vi "DAQmx task start-Pockels modulation AO.vi"(8 "error in (no error)":errorcluster, 11 "Pockels modulation AO task in":refnum<k21>) -> (0 "error out":errorcluster, 3 "Pockels modulation AO task out":refnum<k21>)   [LabVIEW 2020]
uses:
  Globals/gl_Pockels control globals.vi
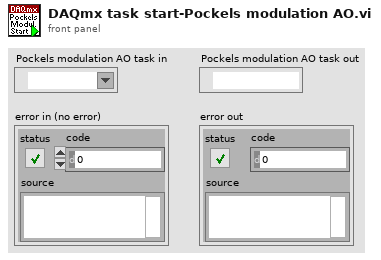
[diagram p1: front panel]
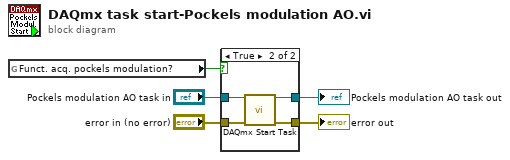
[diagram p0: block diagram]
diagram:
  n1 = global read "gl_Pockels control globals.vi" "Funct. acq. pockels modulation?"() -> (w4:bool)
  n2 = case shown="True" w4 {
    tunnel: [w6 w10] -> w1
    tunnel: [_ w9] -> w2
    tunnel: "error in (no error)" -> [_ w8]
    tunnel: "Pockels modulation AO task in" -> [w6 w7]
    frame False {
    }
    frame True {
      n3 = call <vilib>:"DAQmx Start Task.vi"("task/channels in"=w7, "error in"=w8) -> ("task out"=w10:refnum<k21>, "error out"=w9:errorcluster)  [unwired: 12 in]
    }
  }
  "error out" <- w2
  "Pockels modulation AO task out" <- w1
